vi "Rx FIFOs.vi"(0 "rx.fifo":refnum<k21>, 1 "rx.data sink":enum16{"SFP Port 0", "SFP Port 1", "Host"}(ring)=enum."SFP Port 1", 5 "rx.host fifo":refnum<k21>, 7 "rx.sfp fifo":refnum<k21>) -> ()   [LabVIEW 2016]
uses:
  <vilib>/rvi/DataTransferAndStorage/Container/XNode/niFpgaContainer.xnode
  <vilib>/rvi/FIFO/Fifo_Resource/niFpgaFifoEmulationRefIn.vi
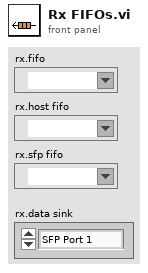
[diagram p1: front panel]
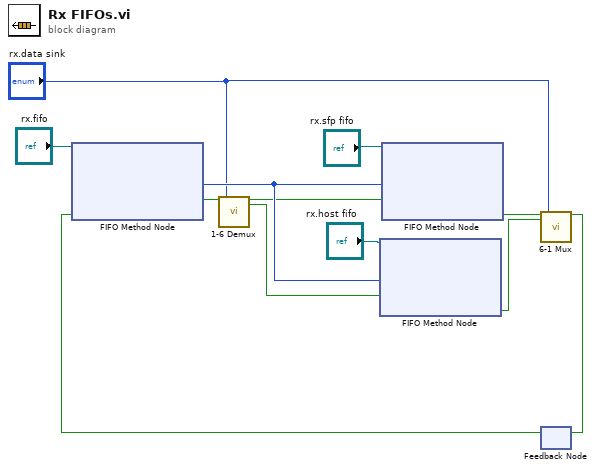
[diagram p0: block diagram]
diagram:
  n1 = feedback #1() -> (w9:bool)  [unwired: 1 in]
  n2 = xnode ("FIFO Method Node")("Ready for Output"=w9, "FIFO In"="rx.fifo") -> ("Element"=w12:u32, "Output Valid"=w11:bool)  [unwired: 1 out]
  n3 = call "1-6 Demux.vi"("input"=w11, "select"="rx.data sink") -> ("output 0"=w4:bool, "output 1"=w3:bool)  [unwired: 12 in, 4 out]
  n4 = xnode ("FIFO Method Node")("Element"=w12, "Input Valid"=w3, "FIFO In"="rx.host fifo") -> ("Ready for Input"=w1:bool)  [unwired: 1 out]
  n5 = xnode ("FIFO Method Node")("Element"=w12, "Input Valid"=w4, "FIFO In"="rx.sfp fifo") -> ("Ready for Input"=w2:bool)  [unwired: 1 out]
  n6 = call "6-1 Mux.vi"("input 0"=w2, "input 1"=w1, "select"="rx.data sink") -> ("output"=w10:bool)  [unwired: 16 in]
  n7 = feedback-in #1(w10) -> ()
